vi "whileloop.vi"() -> ()   [LabVIEW 2021]
panel:
  out "Numeric 2":i32
  out "Numeric":i32
  in  "Stop":bool
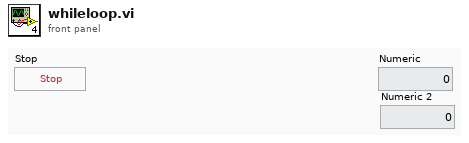
[diagram p1: front panel]
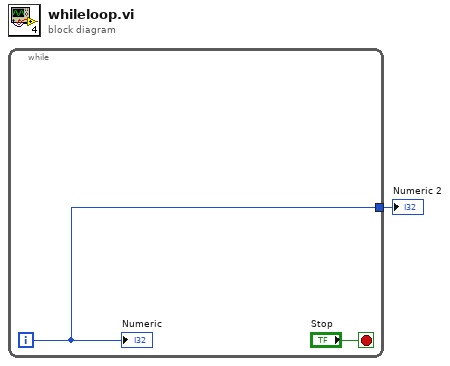
[diagram p0: block diagram]
diagram:
  n1 = while {
    tunnel: [w2] -> w1
    i -> [w2]
    stop <- "Stop" stop-if-true
    "Numeric" <- w2
  }
  "Numeric 2" <- w1
